vi "linear interp iiii- real - z-omega.vi"(0 "z":dbl[](array[numeric]), 5 "omega":dbl[](array[numeric]), 9 "point":dbl, 11 "center":i32=-1) -> (2 "directed sigma":dbl, 3 "directed sigma - abs":dbl, 4 "z out":dbl[](array[numeric]), 6 "omega out":dbl[](array[numeric]), 8 "left":dbl, 10 "center":dbl, 12 "intercept":dbl, 13 "slope":dbl, 14 "value":dbl, 15 "right":dbl)   [LabVIEW 2014]
uses:
  <vilib>/Analysis/baseanly.llb/Real A x B.vi
  Q - not nan -- real.vi
  Q - not nan -- integer.vi
  <vilib>/Analysis/baseanly.llb/Real Inverse Matrix.vi
  <vilib>/Analysis/Matrix/Numeric/Conversions/Array To Matrix - RA2.vi
  <vilib>/Analysis/NI_AALBase.lvlib
  <vilib>/Analysis/Matrix/NI_Matrix.lvlib
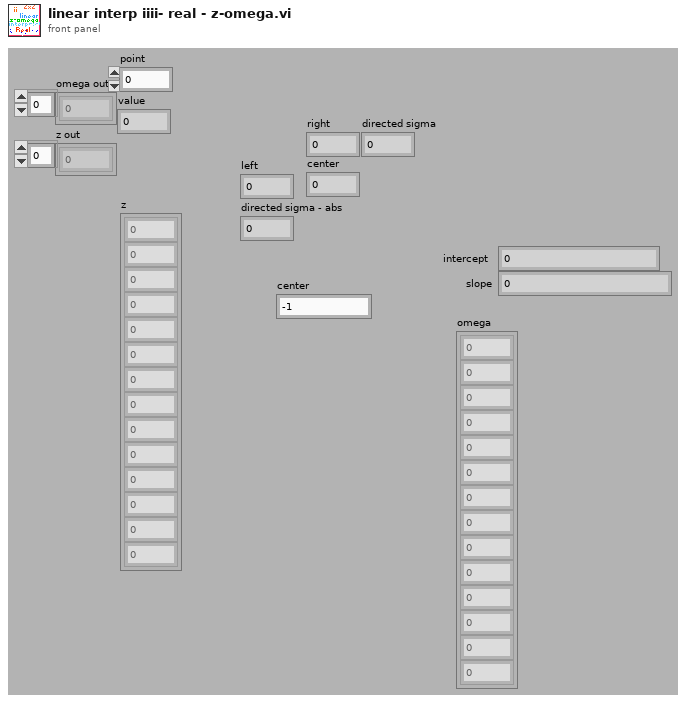
[diagram p1: front panel]
types:
  T1 = typedef "NI_Matrix.lvlib/RealMatrix.ctl" = dbl[][]
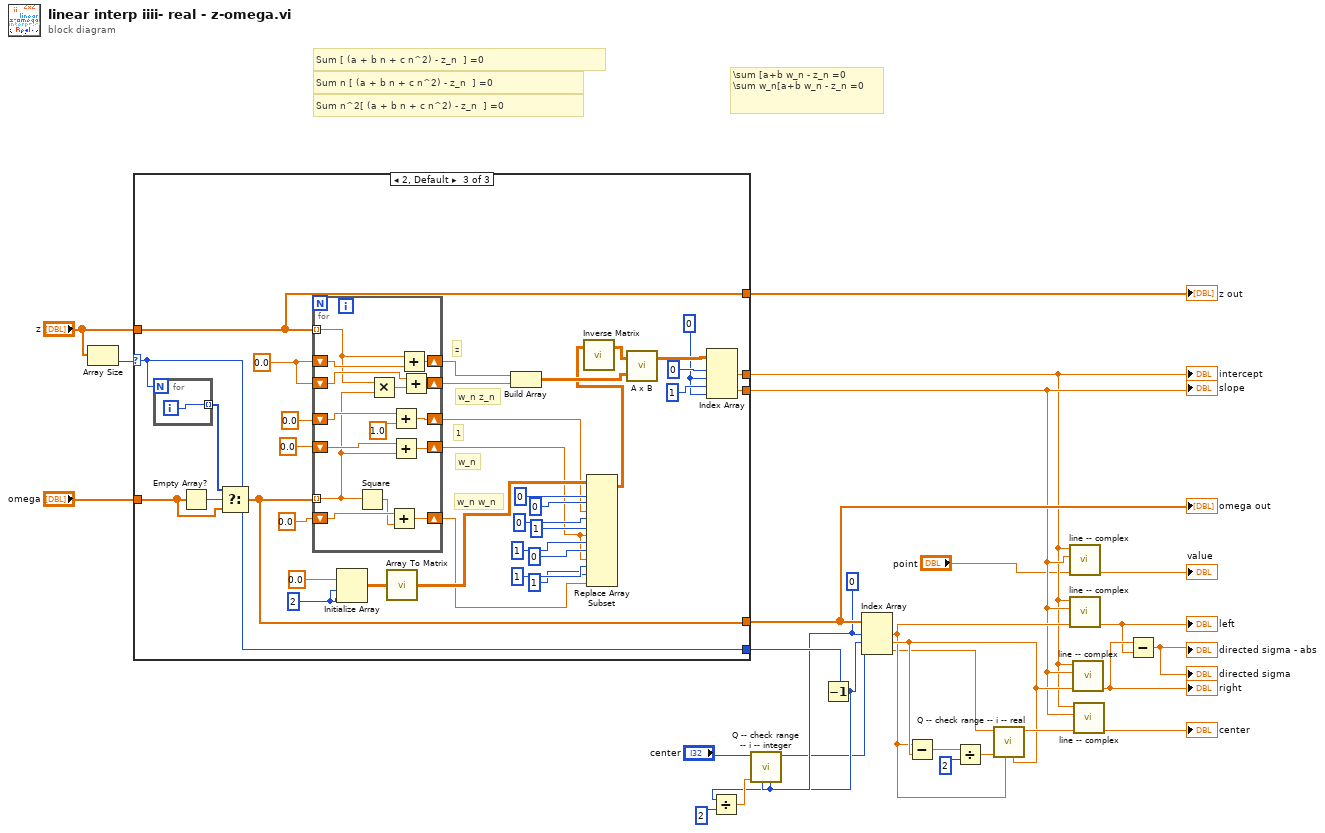
[diagram p0: block diagram]
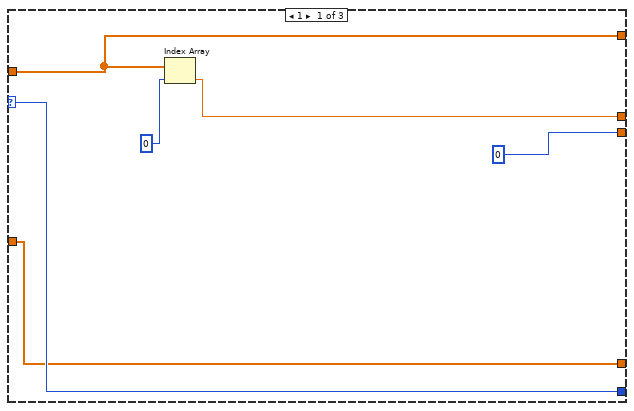
[diagram p2: hidden frame]
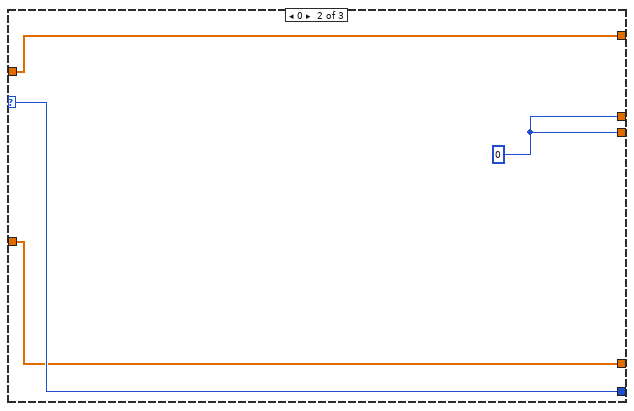
[diagram p3: hidden frame]
diagram:
  w8 = 0 ("n")
  # "\\sum [a+b w_n - z_n =0 \n\\sum w_n[a+b w_n - z_n =0"
  # "Sum n^2[ (a + b n + c n^2) - z_n  ] =0"
  # "Sum n [ (a + b n + c n^2) - z_n  ] =0"
  # "Sum [ (a + b n + c n^2) - z_n  ] =0"
  n1 = Array Size(array="z") -> (size(s)=w19:i32)
  n2 = case shown="2, Default" w19 {
    selector: w19 -> [w31 w37 w62]
    tunnel: [w32 w36 w64] -> w4
    tunnel: [0 ("index") w36 w63] -> w5
    tunnel: "z" -> [w28 w35 w38]
    tunnel: [w31 w37 w62] -> w21
    tunnel: "omega" -> [w29 w34 w60]
    tunnel: [w29 w34 w39] -> w17
    tunnel: [w28 w35 w38] -> w16
    frame 1 {
      n3 = Index Array(array=w28, index=0) -> (element=w32:dbl)
    }
    frame 0 {
      w36 = 0 ("index")
    }
    frame 2, Default {
      w58 = 2 ("n")
      w65 = 0 ("index (row)")
      w72 = 0.0
      # "w_n w_n"
      # "w_n"
      # "1"
      # "w_n z_n"
      # "z"
      n4 = for {
        N: w62 -> [_]
        tunnel: [w74] -> w59 mode=indexing
        i -> [w74]
      }
      n5 = Empty Array?(array=w60) -> (empty?=w61:bool)
      n6 = Select(t=w59, s=w61, f=w60) -> (s? t:f=w39:dbl[])
      n7 = for {
        tunnel: w38 -> [w84] mode=indexing
        shift-right: [w89] -> w71
        shift-left: w72 -> [w88]
        shift-right: [w86] -> w70
        shift-left: w72 -> [w85]
        shift-right: [w82] -> w48
        shift-left: 0.0 -> [w83]
        shift-right: [w79] -> w43
        shift-left: 0.0 -> [w80]
        tunnel: w39 -> [w76] mode=indexing
        shift-right: [w77] -> w42
        shift-left: 0.0 -> [w78]
        n8 = Square(x=w76) -> (x^2=w75:dbl)
        n9 = Multiply(x=w84, y=w76) -> (x*y=w87:dbl)
        n10 = Add(x=w78, y=w75) -> (x+y=w77:dbl)
        n11 = Add(x=w83, y=1.0) -> (x+y=w82:dbl)
        n12 = Add(x=w80, y=w76) -> (x+y=w79:dbl)
        n13 = Add(x=w84, y=w88) -> (x+y=w89:dbl)
        n14 = Add(x=w85, y=w87) -> (x+y=w86:dbl)
      }
      n15 = Initialize Array(0.0 ("n"), w58, w58) -> (w52:dbl[][])
      n16 = call-poly <vilib>:"Array To Matrix.vi"("Real 2D Array"=w52) -> ("Real Matrix"=w57:T1)
      n17 = Build Array(w71, w70) -> (w69:T1)
      n18 = Replace Array Subset(array=w57, new element #1=w48, index (row) #1=0 ("n"), index (col) #1=0 ("n"), new element #2=w43, index (row) #2=0 ("n"), index (col) #2=1 ("n"), new element #3=w43, index (row) #3=1 ("n"), index (col) #3=0 ("n"), new element #4=w42, index (row) #4=1 ("n"), index (col) #4=1 ("n")) -> (w41:T1)
      n19 = call-poly <vilib>:"Inverse Matrix.vi"("Input Matrix"=w41) -> ("Inverse Matrix"=w40:T1)  [unwired: 1 in, 1 out]
      n20 = call-poly <vilib>:"A x B.vi"("B"=w69, "A"=w40) -> ("A x B"=w68:T1)  [unwired: 1 out]
      n21 = Index Array(array=w68, index (row) #1=0 ("index (row)"), index (col) #1=w65, index (row) #2=1 ("index (row)"), index (col) #2=w65) -> (element #1=w64:dbl, element #2=w63:dbl)
    }
  }
  "slope" <- w5
  "intercept" <- w4
  "omega out" <- w17
  "z out" <- w16
  n22 = Decrement(x=w21) -> (x-1=w7:i32)
  n23 = Divide(x=w7, y=2 ("n")) -> (x/y=w10:dbl)
  n24 = call "Q -- check range -- i -- integer.vi"("upper"=w7, "lower"=w8, "default"=w10, "number"="center") -> ("number in range"=w6:i32)  [unwired: 5 in, 2 out]
  n25 = Index Array(array=w17, index #1=w8, index #2=w7, index #3=w6) -> (element #1=w14:dbl, element #2=w15:dbl, element #3=w12:dbl)
  n26 = Subtract(x=w14, y=w15) -> (x-y=w13:dbl)
  n27 = Divide(x=w13, y=2 ("n")) -> (x/y=w22:dbl)
  n28 = call "Q -- check range -- i -- real.vi"("upper"=w15, "lower"=w14, "default"=w22, "number"=w12) -> ("number in range"=w26:dbl)  [unwired: 5 in, 2 out]
  n29 = call "line -- complex.vi"("n"="point", "slope"=w5, "intercept"=w4) -> ("value"=→"value":cdb)  [unwired: 7 in, 1 out]
  n30 = call "line -- complex.vi"("n"=w14, "slope"=w5, "intercept"=w4) -> ("value"=w23:cdb)  [unwired: 7 in, 1 out]
  "left" <- w23
  n31 = call "line -- complex.vi"("n"=w15, "slope"=w5, "intercept"=w4) -> ("value"=w24:cdb)  [unwired: 7 in, 1 out]
  "right" <- w24
  n32 = call "line -- complex.vi"("n"=w26, "slope"=w5, "intercept"=w4) -> ("value"=→"center":cdb)  [unwired: 7 in, 1 out]
  n33 = Subtract(x=w24, y=w23) -> (x-y=→"directed sigma - abs" →"directed sigma":cdb)
